vi "Edit Existing Devices.vi"() -> ()   [LabVIEW 2024, in "User Interface.lvlib"]
uses:
  User Interface.lvlib
  Support/General Type Defs/Edit Devices States.ctl
  Support/General Type Defs/Device Data.ctl
  Support/General Type Defs/Device OS.ctl
  <vilib>/Utility/miscctls.llb/LVRowAndColumnTypeDef.ctl
  Support/General Type Defs/Global Data.vi
  Support/General Type Defs/General Type Definitions.lvlib
panel:
  in  "Alias":string
  in  "Delete":bool
  in  "Update Device":bool
  in  "Device Data":T1
  out "Enum":T3
  out "Existing Devices Table":string[][](table)
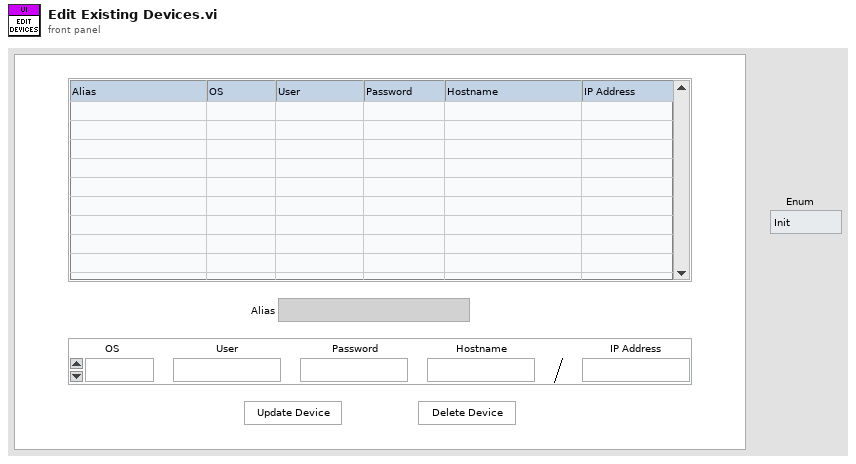
[diagram p1: front panel]
types:
  T1 = typedef "General Type Definitions.lvlib/Device Data.ctl" = cluster{"OS":T2, "User":string, "Password":string, "Hostname":string, "IP Address":string}
  T2 = typedef "General Type Definitions.lvlib/Device OS.ctl" = enum16{"Windows", "Linux"}
  T3 = typedef "General Type Definitions.lvlib/Edit Devices States.ctl" = enum16{"Init", "IDLE", "Display Selection", "Clean Selection", "Delete", "Update", "STOP"}
  T4 = typedef "LVRowAndColumnTypeDef.ctl" = cluster{"Row":i32, "Column":i32}
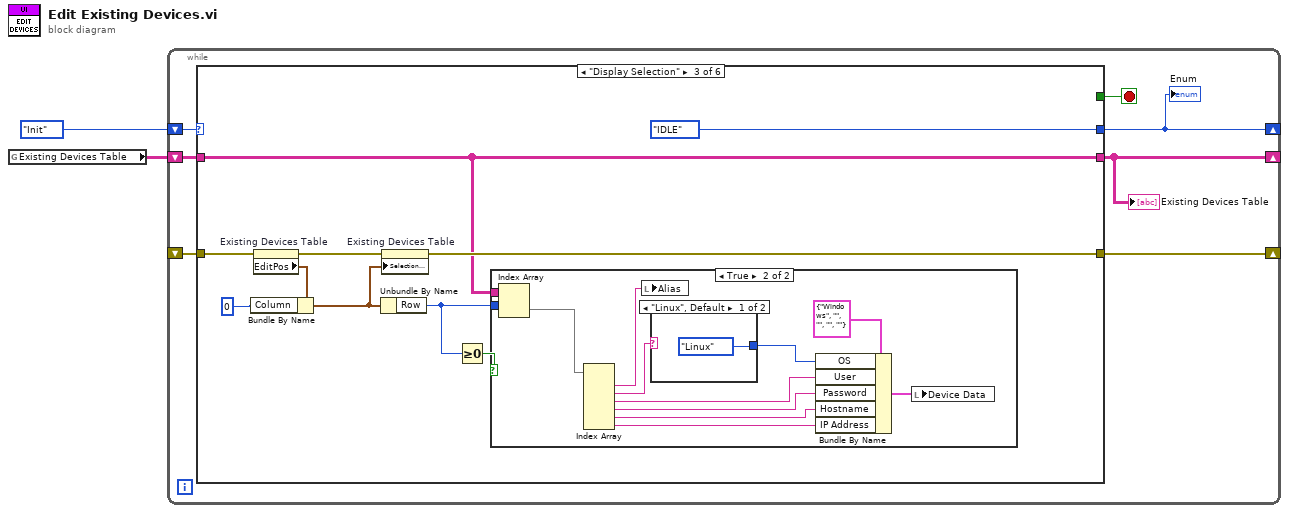
[diagram p0: block diagram]
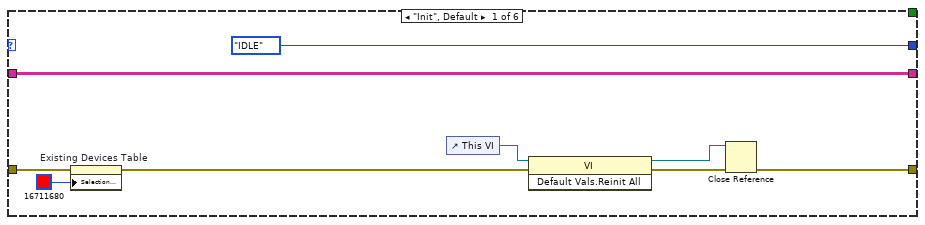
[diagram p2: hidden frame]
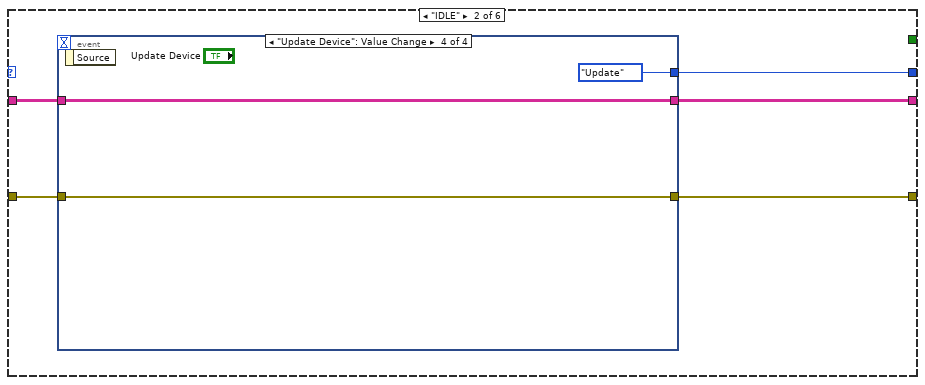
[diagram p3: hidden frame]
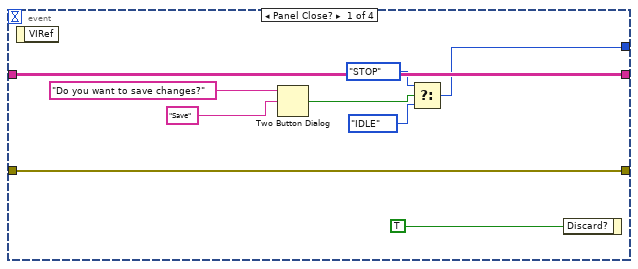
[diagram p4: hidden frame]
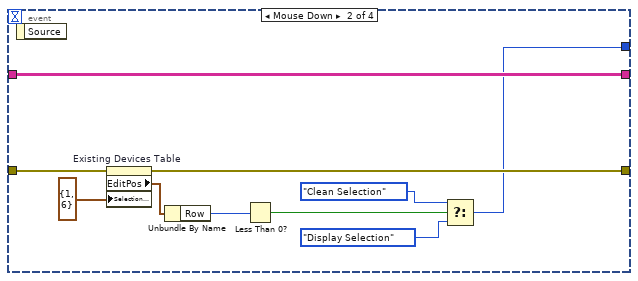
[diagram p5: hidden frame]
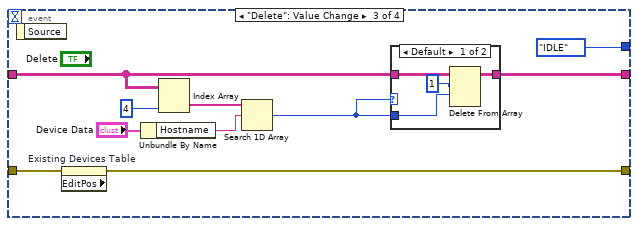
[diagram p6: hidden frame]
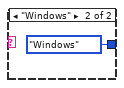
[diagram p9: hidden frame]
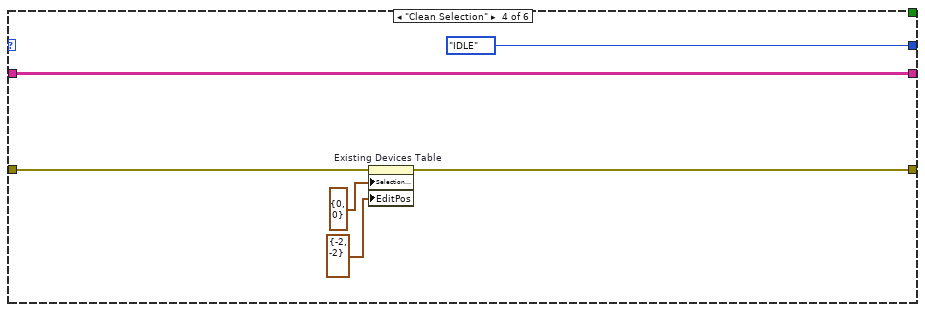
[diagram p10: hidden frame]
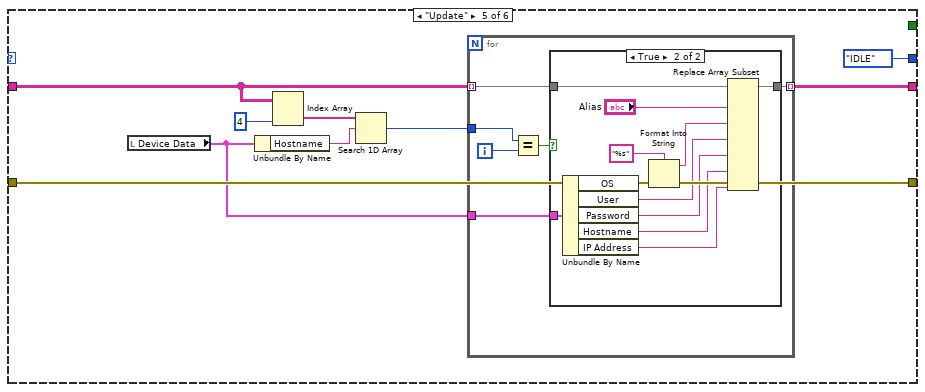
[diagram p11: hidden frame]
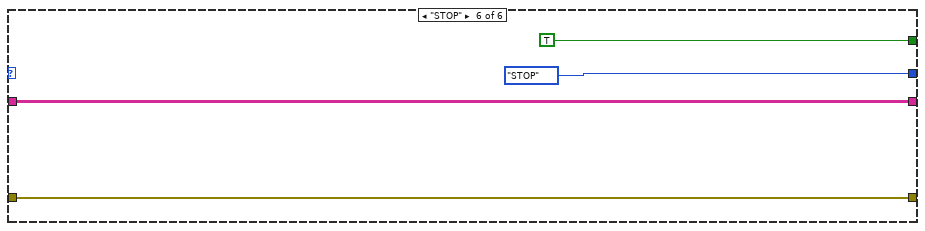
[diagram p13: hidden frame]
diagram:
  n1 = global read "Global Data.vi" "Existing Devices Table"() -> (w1:string[][])
  n2 = while {
    shift-right: [w3] -> _
    shift-left: Edit_Devices_States."Init" -> [w9]
    shift-right: [w7] -> _
    shift-left: w1 -> [w8]
    shift-right: [w5] -> _
    shift-left: _ -> [w4]
    stop <- w6 stop-if-true
    n3 = case shown="\"Display Selection\"" w9 {
      tunnel: w8 -> [w18 w23 w64 w90 w94 w121]
      tunnel: [w18 w22 w64 w90 w92 w121] -> w7
      tunnel: [Edit_Devices_States."IDLE" w21 Edit_Devices_States."IDLE" Edit_Devices_States."IDLE" Edit_Devices_States."IDLE" Edit_Devices_States."STOP"] -> w3
      tunnel: [_ _ _ _ _ TRUE] -> w6
      tunnel: [w10 w19 w65 w87 w95 w118] -> w5
      tunnel: w4 -> [w15 w20 w68 w86 w95 w118]
      frame "Init", Default {
        n4 = property on="Existing Devices Table" class="Tbl (strict)"(error in=w15, "Selection Color"=u32 16711680) -> (error out=w11:errorcluster)  [unwired: 1 in, 1 out]
        n5 = control-ref of="This VI"() -> (w14:refnum<vi>)
        n6 = invoke class="VI" method="Default Vals.Reinit All"(reference=w14, error in=w11) -> (reference out=w12:refnum<vi>, error out=w13:errorcluster)  [unwired: 1 in, 1 out]
        n7 = Close Reference(reference=w12, error in (no error)=w13) -> (error out=w10:errorcluster)
      }
      frame "IDLE" {
        n8 = event shown="[3] \"Update Device\": Value Change" {
          selector: _ -> [_ _ _ _]
          dyn-events: _ -> [_ _ _ _]
          timeout: _ -> [_ _ _ _]
          tunnel: w23 -> [w32 w42 w49 w60]
          tunnel: [w32 w42 w50 w60] -> w22
          tunnel: [w25 w34 Edit_Devices_States."IDLE" Edit_Devices_States."Update"] -> w21
          tunnel: w20 -> [w24 w41 w52 w59]
          tunnel: [w24 w40 w51 w59] -> w19
          event Panel Close? {
            n9 = event-data() -> ()  [unwired: 1 in, 1 out]
            n10 = Two Button Dialog(message="Do you want to save changes?", 2:"Save" ("T button name (\"OK\")")) -> (T button?=w28:bool)  [unwired: 1 in]
            n11 = Select(t=Edit_Devices_States."STOP", s=w28, f=Edit_Devices_States."IDLE") -> (s? t:f=w25:T3)
            n12 = event-data("Discard?"=TRUE) -> ()  [unwired: 1 in, 1 out]
          }
          event Mouse Down {
            n13 = event-data() -> ()  [unwired: 1 in, 1 out]
            n14 = property on="Existing Devices Table" class="Tbl (strict)"(error in=w41, "Selection Size"=T4 {"Row"=1, "Column"=6}) -> (error out=w40:errorcluster, "EditPos"=w36:T4)  [unwired: 1 in, 1 out]
            n15 = Unbundle By Name(w36) -> ("Row"=w33:i32)
            n16 = Less Than 0?(x=w33) -> (x < 0?=w39:bool)
            n17 = Select(t=Edit_Devices_States."Clean Selection", s=w39, f=Edit_Devices_States."Display Selection") -> (s? t:f=w34:T3)
          }
          event "Delete": Value Change {
            n18 = event-data() -> ()  [unwired: 1 in, 1 out]
            n19 = property on="Existing Devices Table" class="Tbl (strict)" props=["EditPos"](error in=w52) -> (error out=w51:errorcluster)  [unwired: 1 in, 2 out]
            n20 = Unbundle By Name("Device Data") -> ("Hostname"=w45:string)
            n21 = Index Array(array=w49, index (col)=4) -> (element=w46:string[])  [unwired: 1 in]
            n22 = Search 1D Array(1D array=w46, element=w45) -> (index of element=w44:i32)  [unwired: 1 in]
            n23 = case shown="Default" w44 {
              tunnel: [w55 w57] -> w50
              tunnel: w49 -> [w54 w57]
              tunnel: w44 -> [w53 _]
              frame Default {
                n24 = Delete From Array(array=w54, length=1, index (row)=w53) -> (array with subset deleted=w55:string[][])  [unwired: 1 in, 1 out]
              }
              frame -1 {
              }
            }
          }
          event "Update Device": Value Change {
            n25 = event-data() -> ()  [unwired: 1 in, 1 out]
          }
        }
      }
      frame "Display Selection" {
        n26 = property on="Existing Devices Table" class="Tbl (strict)"(error in=w68) -> (error out=w66:errorcluster, "EditPos"=w67:T4)  [unwired: 1 in, 1 out]
        n27 = Bundle By Name(cluster=w67, "Column"=0) -> (w63:T4)
        n28 = Unbundle By Name(w63) -> ("Row"=w61:i32)
        n29 = property on="Existing Devices Table" class="Tbl (strict)"(error in=w66, "Selection Start"=w63) -> (error out=w65:errorcluster)  [unwired: 1 in, 1 out]
        n30 = Greater Or Equal To 0?(x=w61) -> (x >= 0?=w62:bool)
        n31 = case shown="True" w62 {
          tunnel: w64 -> [_ w82]
          tunnel: w61 -> [_ w81]
          frame False {
          }
          frame True {
            n32 = Index Array(array=w82, index (row)=w81) -> (element=w73:string[])  [unwired: 1 in]
            n33 = Index Array(array=w73) -> (element #1=w71:string, element #2=w76:string, element #3=w77:string, element #4=w80:string, element #5=w79:string, element #6=w78:string)  [unwired: 6 in]
            n34 = local write "Alias"(w71) -> ()
            n35 = case shown="\"Linux\", Default" w76 {
              tunnel: [Device_OS."Linux" ("OS") Device_OS."Windows" ("OS")] -> w75
              frame "Linux", Default {
              }
              frame "Windows" {
              }
            }
            n36 = Bundle By Name(cluster=T1 {"OS"=enum."Windows", "User"="", "Password"="", "Hostname"="", "IP Address"=""} ("Device Data"), "OS"=w75, "User"=w77, "Password"=w80, "Hostname"=w79, "IP Address"=w78) -> (w72:T1)
            n37 = local write "Device Data"(w72) -> ()
          }
        }
      }
      frame "Clean Selection" {
        n38 = property on="Existing Devices Table" class="Tbl (strict)"(error in=w86, "Selection Size"=T4 {"Row"=0, "Column"=0}, "EditPos"=T4 {"Row"=-2, "Column"=-2} ("Edit Position")) -> (error out=w87:errorcluster)  [unwired: 1 in, 1 out]
      }
      frame "Update" {
        n39 = local read "Device Data"() -> (w91:T1)
        n40 = Unbundle By Name(w91) -> ("Hostname"=w98:string)
        n41 = Index Array(array=w94, index (col)=4) -> (element=w99:string[])  [unwired: 1 in]
        n42 = Search 1D Array(1D array=w99, element=w98) -> (index of element=w93:i32)  [unwired: 1 in]
        n43 = for {
          tunnel: w94 -> [w102] mode=indexing
          tunnel: w93 -> [w104]
          tunnel: [w101] -> w92 mode=indexing
          tunnel: w91 -> [w100]
          i -> [w105]
          n44 = Equal?(x=w104, y=w105) -> (x = y?=w103:bool)
          n45 = case shown="True" w103 {
            tunnel: w102 -> [w106 w117]
            tunnel: [w106 w116] -> w101
            tunnel: w100 -> [_ w115]
            frame False {
            }
            frame True {
              n46 = Unbundle By Name(w115) -> ("OS"=w114:T2, "User"=w111:string, "Password"=w110:string, "Hostname"=w109:string, "IP Address"=w108:string)
              n47 = Format Into String(format string="%s", w114) -> (resulting string=w112:string)  [unwired: 2 in, 1 out]
              n48 = Replace Array Subset(array=w117, new element #1="Alias", new element #2=w112, new element #3=w111, new element #4=w110, new element #5=w109, new element #6=w108) -> (w116:string[])  [unwired: 6 in]
            }
          }
        }
      }
      frame "STOP" {
      }
    }
    "Existing Devices Table" <- w7
    "Enum" <- w3
  }
